vi "fix supported types and targets.vi"(8 "error in":errorcluster, 10 "decideprojectfeatures in":refnum<class "DecideModuleFeatures.lvclass">, 11 "user project in":refnum<vi>) -> (0 "error out":errorcluster, 3 "user project out":refnum<vi>)   [LabVIEW 2013, in "DecideModuleFeatures.lvclass"]
uses:
  DecideModuleFeatures.lvclass
  DecideModuleFeatures.lvclass/DecideModuleFeatures.ctl
  Read supported data types.vi
  Read supported targets.vi
  Read instances allowed.vi
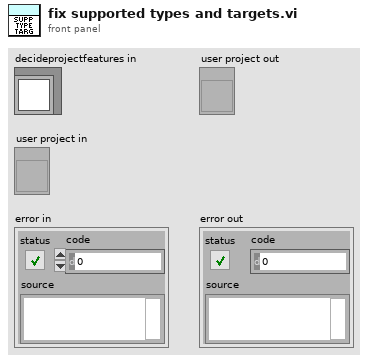
[diagram p1: front panel]
types:
  T1 = typedef "tag bus.lvlib/tag descriptor.lvclass/Data Type.ctl" = enum16{"Double", "Single", "I64", "I32", "I16", "I8", "U64", "U32", "U16", "U8", "Boolean", "String", "Array of Double", "Array of Single", "Array of I64", "Array of I32", "Array of I16", "Array of I8", "Array of U64", "Array of U32", "Array of U16", "Array of U8", "Array of Boolean", "Array of String"}
  T2 = typedef "TBM configuration.lvclass/Target Types.ctl" = enum16{"Windows", "Mac", "Linux", "Linux RT ARM", "VxWorks", "Pharlap", "Other", "Linux RT x64"}
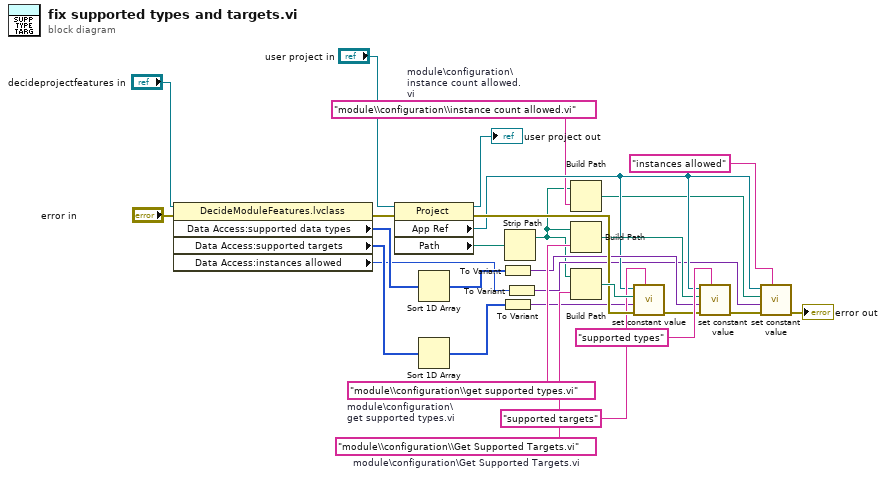
[diagram p0: block diagram]
diagram:
  w5 = "module\\configuration\\instance count allowed.vi"  # module\configuration\instance count allowed.vi
  w24 = "module\\configuration\\get supported types.vi"  # module\configuration\get supported types.vi
  w25 = "module\\configuration\\Get Supported Targets.vi"  # module\configuration\Get Supported Targets.vi
  n1 = property class="DecideModuleFeatures.lvclass"(reference="decideprojectfeatures in", error in="error in") -> (error out=w21:errorcluster, "Data Access:supported data types"=w19:T1[], "Data Access:supported targets"=w20:T2[], "Data Access:instances allowed"=w7:i32)  [unwired: 1 out]
  n2 = property class="Project"(reference="user project in", error in=w21) -> (reference out=→"user project out":refnum<vi>, error out=w26:errorcluster, "App Ref"=w10:refnum<vi>, "Path"=w4:path)
  n3 = Sort 1D Array(array=w19) -> (sorted array=w12:T1[])
  n4 = Sort 1D Array(array=w20) -> (sorted array=w11:T2[])
  n5 = To Variant(anything=w12) -> (Variant=w14:variant)
  n6 = To Variant(anything=w11) -> (Variant=w17:variant)
  n7 = Strip Path(path=w4) -> (stripped path=w1:path)  [unwired: 1 out]
  n8 = To Variant(anything=w7) -> (Variant=w6:variant)
  n9 = Build Path(base path=w1, name or relative path=w5) -> (appended path=w3:path)
  n10 = Build Path(base path=w1, name or relative path=w24) -> (appended path=w13:path)
  n11 = Build Path(base path=w1, name or relative path=w25) -> (appended path=w27:path)
  n12 = call "set constant value.vi"("control name"="supported targets" ("y"), "error in"=w26, "data to set"=w17, "vi path"=w27, "application in"=w10) -> ("error out"=w15:errorcluster)  [unwired: 6 in]
  n13 = call "set constant value.vi"("control name"="supported types" ("y"), "error in"=w15, "data to set"=w14, "vi path"=w13, "application in"=w10) -> ("error out"=w9:errorcluster)  [unwired: 6 in]
  n14 = call "set constant value.vi"("control name"="instances allowed", "error in"=w9, "data to set"=w6, "vi path"=w3, "application in"=w10) -> ("error out"=→"error out":errorcluster)  [unwired: 6 in]
